vi "Test Read-Write Control.vi"(8 "error in (no error)":errorcluster) -> (0 "error out":errorcluster, 3 "Pass?":bool)   [LabVIEW 2020]
uses:
  G-Unicode/Types/UTF-8 String/UTF-8 String.lvclass/UTF-8 String.ctl
  d7f44957-dd1e-4aab-aae7-486b9bf0438c.vi
  1da8a88b-ae4e-476f-a58c-12139bd44ca5.vi
  11ce0e2c-e1a8-46a3-af78-7df26efc8245.vi
  3b8e0032-af78-4c0b-9bbb-79828ff8a6dd.vi
  70f15325-3570-4740-90b7-b159886a8434.vi
  c5b5f753-7993-4590-ab7a-38cd070e680f.vi
  1ceb00d4-36f5-49cb-928e-534e3e1f0591.vi
  1e068905-1677-418d-bf6d-609c6dcf122f.vi
  d87d6912-68ee-4c4f-8e1f-9eaf2c3e8737.vi
  8bfd12a5-a12f-46b2-9c2c-ba6b48562335.vi
  faa5ed0a-1e2a-49a9-b47c-7d87d0d78869.vi
  b51df372-b908-46a9-9cd9-1bce9bcba761.vi
  c50d1312-50c6-48d3-b875-d8e2e1e6006d.vi
  0f0a57d2-251a-4010-ac87-403ca3d19de3.vi
  3f50c59c-438d-4159-8265-e7e5e4819d1d.vi
  63b695b2-ee1d-4cc0-8b09-8d83892ddc19.vi
  a0d048c9-5e62-40e8-86eb-582b39f8129a.vi
  f481c7ac-37a4-4879-9d59-93dd94c77838.vi
  a84f4c8b-19ca-4313-b3c0-0071757116b8.vi
  daac9e31-94d2-45d0-adb4-e535b058ebe1.vi
  2abff34c-ba54-40bb-bfb0-e7a9eb1a66c8.vi
  258a67cf-78bc-49d9-a232-fa9eda3d4c17.vi
  843d702d-5434-496e-8b84-06685370aefe.vi
  b9bba32d-5ca2-4258-b841-0da24b58b874.vi
  aa946967-5c50-4c02-a82c-9d1d96941c38.vi
  74cd828c-e59a-47d5-9363-431a13b30ca9.vi
  4c20338b-6e60-4a75-91ad-9e96f58f92b0.vi
  d7f44957-dd1e-4aab-aae7-486b9bf0438c.vi/5206cb6b-04fb-41f5-a37e-29c14f142303.vi
  1da8a88b-ae4e-476f-a58c-12139bd44ca5.vi/394fe735-5a0a-4c6e-b10c-ef5f4bad8cdd.vi
  1da8a88b-ae4e-476f-a58c-12139bd44ca5.vi/c6ff4536-5c5f-4898-b0f4-ba79e0235d06.vi
  11ce0e2c-e1a8-46a3-af78-7df26efc8245.vi/3a31b270-3bb6-4c58-a256-c5fcc2c98f09.vi
  11ce0e2c-e1a8-46a3-af78-7df26efc8245.vi/0ec5df2d-ef9b-4f84-a6a8-ffcedd45c4dc.vi
  3b8e0032-af78-4c0b-9bbb-79828ff8a6dd.vi/5206cb6b-04fb-41f5-a37e-29c14f142303.vi
  70f15325-3570-4740-90b7-b159886a8434.vi/394fe735-5a0a-4c6e-b10c-ef5f4bad8cdd.vi
  70f15325-3570-4740-90b7-b159886a8434.vi/c6ff4536-5c5f-4898-b0f4-ba79e0235d06.vi
  c5b5f753-7993-4590-ab7a-38cd070e680f.vi/3a31b270-3bb6-4c58-a256-c5fcc2c98f09.vi
  c5b5f753-7993-4590-ab7a-38cd070e680f.vi/0ec5df2d-ef9b-4f84-a6a8-ffcedd45c4dc.vi
  1ceb00d4-36f5-49cb-928e-534e3e1f0591.vi/5206cb6b-04fb-41f5-a37e-29c14f142303.vi
  1e068905-1677-418d-bf6d-609c6dcf122f.vi/394fe735-5a0a-4c6e-b10c-ef5f4bad8cdd.vi
  1e068905-1677-418d-bf6d-609c6dcf122f.vi/c6ff4536-5c5f-4898-b0f4-ba79e0235d06.vi
  d87d6912-68ee-4c4f-8e1f-9eaf2c3e8737.vi/3a31b270-3bb6-4c58-a256-c5fcc2c98f09.vi
  d87d6912-68ee-4c4f-8e1f-9eaf2c3e8737.vi/0ec5df2d-ef9b-4f84-a6a8-ffcedd45c4dc.vi
  8bfd12a5-a12f-46b2-9c2c-ba6b48562335.vi/5206cb6b-04fb-41f5-a37e-29c14f142303.vi
  faa5ed0a-1e2a-49a9-b47c-7d87d0d78869.vi/394fe735-5a0a-4c6e-b10c-ef5f4bad8cdd.vi
  faa5ed0a-1e2a-49a9-b47c-7d87d0d78869.vi/c6ff4536-5c5f-4898-b0f4-ba79e0235d06.vi
  b51df372-b908-46a9-9cd9-1bce9bcba761.vi/3a31b270-3bb6-4c58-a256-c5fcc2c98f09.vi
  b51df372-b908-46a9-9cd9-1bce9bcba761.vi/0ec5df2d-ef9b-4f84-a6a8-ffcedd45c4dc.vi
  c50d1312-50c6-48d3-b875-d8e2e1e6006d.vi/5206cb6b-04fb-41f5-a37e-29c14f142303.vi
  0f0a57d2-251a-4010-ac87-403ca3d19de3.vi/394fe735-5a0a-4c6e-b10c-ef5f4bad8cdd.vi
  0f0a57d2-251a-4010-ac87-403ca3d19de3.vi/c6ff4536-5c5f-4898-b0f4-ba79e0235d06.vi
  3f50c59c-438d-4159-8265-e7e5e4819d1d.vi/3a31b270-3bb6-4c58-a256-c5fcc2c98f09.vi
  3f50c59c-438d-4159-8265-e7e5e4819d1d.vi/0ec5df2d-ef9b-4f84-a6a8-ffcedd45c4dc.vi
  63b695b2-ee1d-4cc0-8b09-8d83892ddc19.vi/5206cb6b-04fb-41f5-a37e-29c14f142303.vi
  a0d048c9-5e62-40e8-86eb-582b39f8129a.vi/394fe735-5a0a-4c6e-b10c-ef5f4bad8cdd.vi
  a0d048c9-5e62-40e8-86eb-582b39f8129a.vi/c6ff4536-5c5f-4898-b0f4-ba79e0235d06.vi
  f481c7ac-37a4-4879-9d59-93dd94c77838.vi/3a31b270-3bb6-4c58-a256-c5fcc2c98f09.vi
  f481c7ac-37a4-4879-9d59-93dd94c77838.vi/0ec5df2d-ef9b-4f84-a6a8-ffcedd45c4dc.vi
  a84f4c8b-19ca-4313-b3c0-0071757116b8.vi/5206cb6b-04fb-41f5-a37e-29c14f142303.vi
  daac9e31-94d2-45d0-adb4-e535b058ebe1.vi/394fe735-5a0a-4c6e-b10c-ef5f4bad8cdd.vi
  daac9e31-94d2-45d0-adb4-e535b058ebe1.vi/c6ff4536-5c5f-4898-b0f4-ba79e0235d06.vi
  2abff34c-ba54-40bb-bfb0-e7a9eb1a66c8.vi/3a31b270-3bb6-4c58-a256-c5fcc2c98f09.vi
  2abff34c-ba54-40bb-bfb0-e7a9eb1a66c8.vi/0ec5df2d-ef9b-4f84-a6a8-ffcedd45c4dc.vi
  258a67cf-78bc-49d9-a232-fa9eda3d4c17.vi/5206cb6b-04fb-41f5-a37e-29c14f142303.vi
  843d702d-5434-496e-8b84-06685370aefe.vi/394fe735-5a0a-4c6e-b10c-ef5f4bad8cdd.vi
  843d702d-5434-496e-8b84-06685370aefe.vi/c6ff4536-5c5f-4898-b0f4-ba79e0235d06.vi
  b9bba32d-5ca2-4258-b841-0da24b58b874.vi/3a31b270-3bb6-4c58-a256-c5fcc2c98f09.vi
  b9bba32d-5ca2-4258-b841-0da24b58b874.vi/0ec5df2d-ef9b-4f84-a6a8-ffcedd45c4dc.vi
  aa946967-5c50-4c02-a82c-9d1d96941c38.vi/5206cb6b-04fb-41f5-a37e-29c14f142303.vi
  74cd828c-e59a-47d5-9363-431a13b30ca9.vi/394fe735-5a0a-4c6e-b10c-ef5f4bad8cdd.vi
  74cd828c-e59a-47d5-9363-431a13b30ca9.vi/c6ff4536-5c5f-4898-b0f4-ba79e0235d06.vi
  4c20338b-6e60-4a75-91ad-9e96f58f92b0.vi/3a31b270-3bb6-4c58-a256-c5fcc2c98f09.vi
  4c20338b-6e60-4a75-91ad-9e96f58f92b0.vi/0ec5df2d-ef9b-4f84-a6a8-ffcedd45c4dc.vi
  G-Unicode/Private/Conversion/Text as Encoded String.vi
  G-Unicode/Private/Conversion/Polymorphic VIs/Text as Encoded String (UTF-8 String).vi
  G-Unicode/Private/Conversion/String as UTF-8 String.vi
  G-Unicode/Private/Conversion/Polymorphic VIs/String as UTF-8 String (LabVIEW String).vi
  G-Unicode/Types/UTF-8 String/Read Encoded UTF-8 String.vi
  G-Unicode/Types/UTF-8 String/New UTF-8 String.vi
  G-Unicode/Private/Conversion/Text to UTF-8.vi
  G-Unicode/Private/Conversion/Polymorphic VIs/Text to UTF-8 (LabVIEW String).vi
  G-Unicode/Private/Conversion/Encoded UTF-8 String to Encoded UTF-16LE String.vi
  G-Unicode/Private/User Interface/Write String.vi
  G-Unicode/Private/User Interface/Read String.vi
  G-Unicode/Unicode/Detect String Encoding.vi
  G-Unicode/Private/Conversion/Encoded UTF-16LE String to Encoded UTF-8 String.vi
  G-Unicode/Private/User Interface/Write String Array (1D).vi
  G-Unicode/Private/User Interface/Read String Array (1D).vi
  G-Unicode/Private/User Interface/Write String Array (2D).vi
  G-Unicode/Private/User Interface/Read String Array (2D).vi
  G-Unicode/Private/User Interface/Write Ring Control.vi
  G-Unicode/Private/User Interface/Read Ring Control.vi
  G-Unicode/Private/User Interface/Write MultCol Listbox Data.vi
  G-Unicode/Private/User Interface/Read MultCol Listbox Data.vi
  G-Unicode/Private/User Interface/Write Listbox Data.vi
  G-Unicode/Private/User Interface/Read Listbox Data.vi
  G-Unicode/Private/User Interface/Write Table Data.vi
  G-Unicode/Private/User Interface/Read Table Data.vi
  G-Unicode/Private/User Interface/Write Tab Control.vi
  G-Unicode/Private/User Interface/Read Tab Control.vi
  G-Unicode/Types/UTF-8 String/UTF-8 String.lvclass
panel:
  in  "Tab Control":enum32{"Page 1", "Page 2", "Page 3", "Page 4"}(tab)
  in  "Multicolumn Listbox":i32(listbox)
  in  "Listbox":i32(listbox)
  in  "Table Control":string[][](table)
  in  "Menu Ring":u16(ring)
  in  "Text Ring":u16(ring)
  in  "String Array (2D)":string[][](array[string])
  in  "String Array (1D)":string[](array[string])
  in  "String":string
  # "Note the dropdowns for the ring controls aren't rendered correctly, but when selected it looks OK."
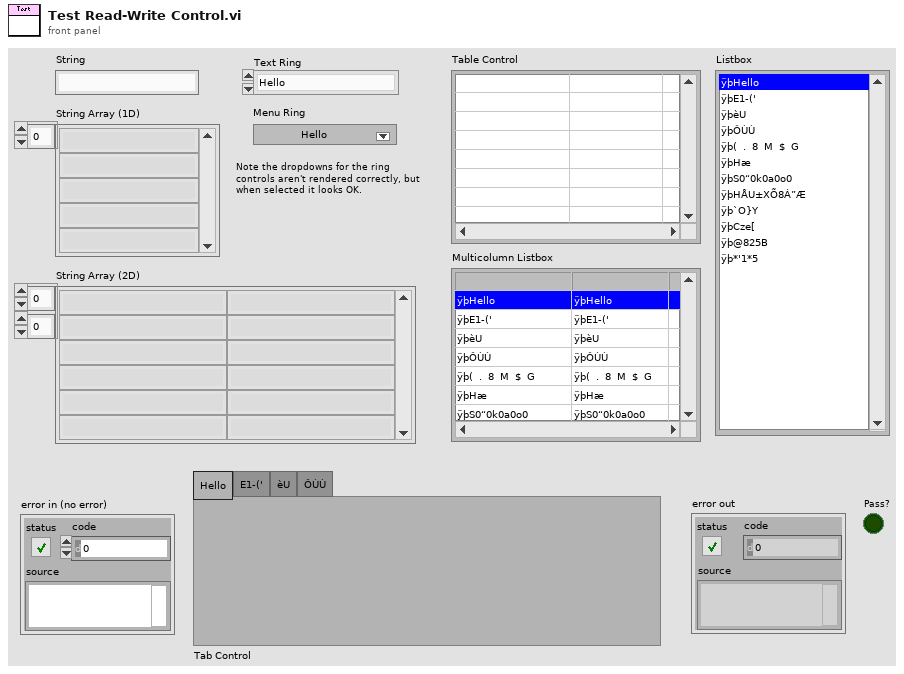
[diagram p1: front panel]
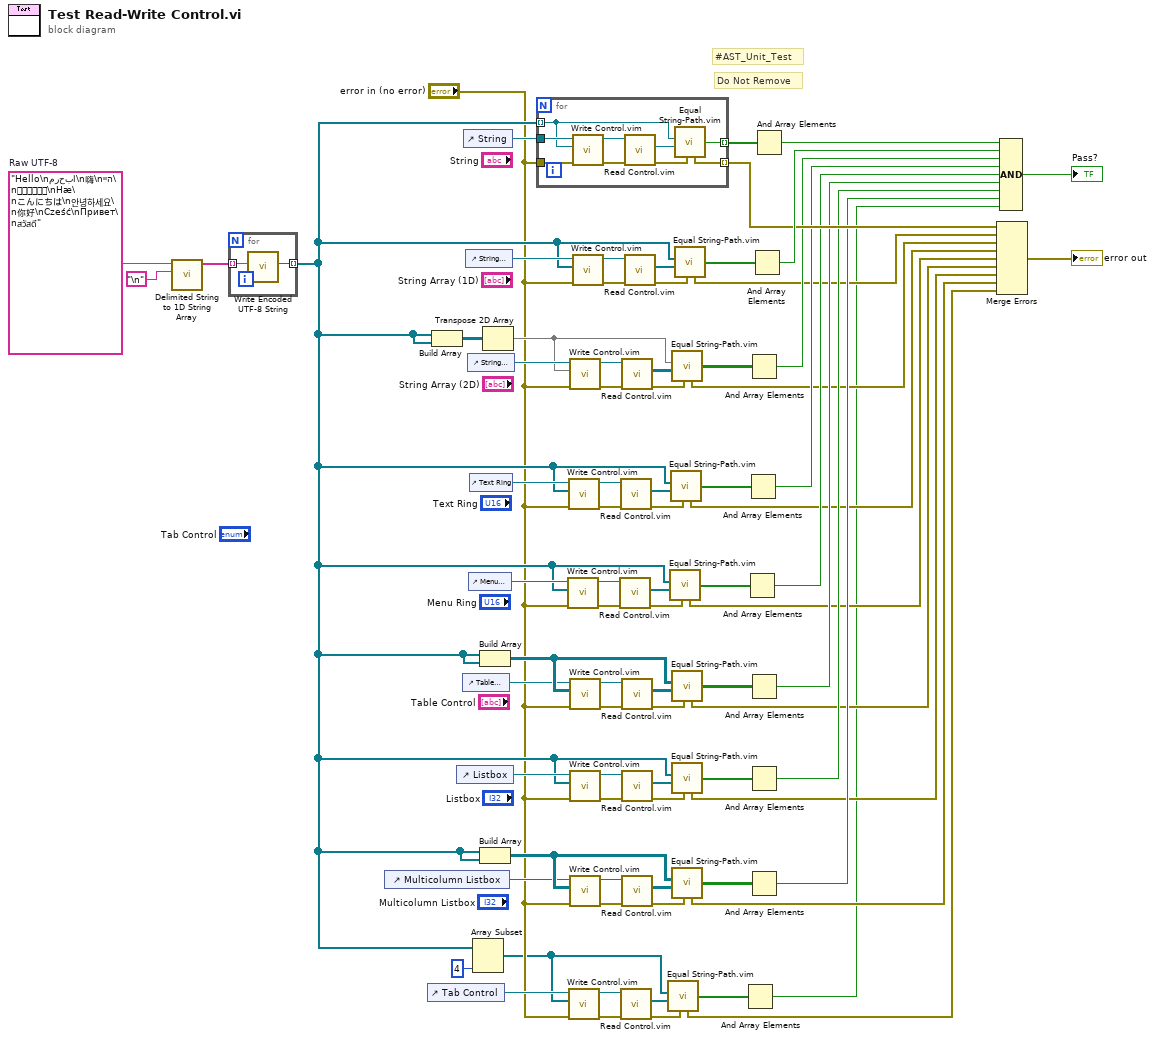
[diagram p0: block diagram]
diagram:
  w80 = "Hello\nمرحبا\n嗨\nהיי\nनमस्ते\nHæ\nこんにちは\n안녕하세요\n你好\nCześć\nПривет\nสวัสดี"  # Raw UTF-8
  # "Do Not Remove"
  # "#AST_Unit_Test"
  n1 = call <vilib>:"Delimited String to 1D String Array.vi"("delimiter"="\n", "delimited string"=w80) -> ("string array"=w79:string[])  [unwired: 9 in]
  n2 = for {
    tunnel: w79 -> [w83] mode=indexing
    tunnel: [w82] -> w12 mode=indexing
    n3 = call "Write Encoded UTF-8 String.vi"("Encoded UTF-8 String"=w83) -> ("UTF-8 String"=w82:refnum<class "UTF-8 String.lvclass">)  [unwired: 10 in]
  }
  n4 = control-ref of="Multicolumn Listbox"() -> (w29:refnum<vi>)
  n5 = control-ref of="Tab Control"() -> (w10:refnum<vi>)
  n6 = Build Array(w12, w12) -> (w62:refnum<class "UTF-8 String.lvclass">[][])
  n7 = control-ref of="Listbox"() -> (w36:refnum<vi>)
  n8 = control-ref of="Table Control"() -> (w42:refnum<vi>)
  n9 = control-ref of="String"() -> (w78:refnum<vi>)
  n10 = control-ref of="String Array (1D)"() -> (w13:refnum<vi>)
  n11 = control-ref of="String Array (2D)"() -> (w63:refnum<vi>)
  n12 = control-ref of="Menu Ring"() -> (w50:refnum<vi>)
  n13 = control-ref of="Text Ring"() -> (w55:refnum<vi>)
  n14 = Array Subset(array=w12, length=4) -> (w6:refnum<class "UTF-8 String.lvclass">[])  [unwired: 1 in]
  n15 = Build Array(w12, w12) -> (w43:refnum<class "UTF-8 String.lvclass">[][])
  n16 = Build Array(w12, w12) -> (w34:refnum<class "UTF-8 String.lvclass">[][])
  n17 = Transpose 2D Array(2D array=w62) -> (transposed array=w60:refnum<class "UTF-8 String.lvclass">[][])
  n18 = for {
    tunnel: w78 -> [w91]
    tunnel: w12 -> [w84] mode=indexing
    tunnel: "error in (no error)" -> [w90]
    tunnel: [w85] -> w68 mode=indexing
    tunnel: [w89] -> w77 mode=indexing
    n19 = call "Write Control.vim"("error in"=w90, "Text"=w84, "Control Ref"=w91) -> ("error out"=w87:errorcluster, "Control Ref dup"=w88:refnum<vi>)  [unwired: 7 in]
    n20 = call "Read Control.vim"("error in"=w87, "Control Ref"=w88) -> ("error out"=w86:errorcluster, "UTF-8 String"=w92:refnum<class "UTF-8 String.lvclass">)  [unwired: 7 in, 1 out]
    n21 = call "Equal String-Path.vim"("error in"=w86, "y"=w92, "x"=w84) -> ("error out"=w85:errorcluster, "Equal?"=w89:bool)  [unwired: 6 in]
  }
  n22 = call "Write Control.vim"("error in"="error in (no error)", "Text"=w12, "Control Ref"=w50) -> ("error out"=w53:errorcluster, "Control Ref dup"=w54:refnum<vi>)  [unwired: 7 in]
  n23 = call "Write Control.vim"("error in"="error in (no error)", "Text"=w12, "Control Ref"=w55) -> ("error out"=w57:errorcluster, "Control Ref dup"=w56:refnum<vi>)  [unwired: 7 in]
  n24 = call "Write Control.vim"("error in"="error in (no error)", "Text"=w6, "Control Ref"=w10) -> ("error out"=w8:errorcluster, "Control Ref dup"=w1:refnum<vi>)  [unwired: 7 in]
  n25 = call "Write Control.vim"("error in"="error in (no error)", "Text"=w60, "Control Ref"=w63) -> ("error out"=w66:errorcluster, "Control Ref dup"=w64:refnum<vi>)  [unwired: 7 in]
  n26 = call "Write Control.vim"("error in"="error in (no error)", "Text"=w43, "Control Ref"=w42) -> ("error out"=w45:errorcluster, "Control Ref dup"=w47:refnum<vi>)  [unwired: 7 in]
  n27 = call "Write Control.vim"("error in"="error in (no error)", "Text"=w12, "Control Ref"=w36) -> ("error out"=w38:errorcluster, "Control Ref dup"=w37:refnum<vi>)  [unwired: 7 in]
  n28 = call "Write Control.vim"("error in"="error in (no error)", "Text"=w34, "Control Ref"=w29) -> ("error out"=w32:errorcluster, "Control Ref dup"=w30:refnum<vi>)  [unwired: 7 in]
  n29 = call "Write Control.vim"("error in"="error in (no error)", "Text"=w12, "Control Ref"=w13) -> ("error out"=w71:errorcluster, "Control Ref dup"=w73:refnum<vi>)  [unwired: 7 in]
  n30 = call "Read Control.vim"("error in"=w53, "Control Ref"=w54) -> ("error out"=w19:errorcluster, "UTF-8 String"=w52:refnum<class "UTF-8 String.lvclass">[])  [unwired: 7 in, 1 out]
  n31 = call "Read Control.vim"("error in"=w57, "Control Ref"=w56) -> ("error out"=w21:errorcluster, "UTF-8 String"=w58:refnum<class "UTF-8 String.lvclass">[])  [unwired: 7 in, 1 out]
  n32 = call "Read Control.vim"("error in"=w8, "Control Ref"=w1) -> ("error out"=w5:errorcluster, "UTF-8 String"=w7:refnum<class "UTF-8 String.lvclass">[])  [unwired: 7 in, 1 out]
  n33 = call "Read Control.vim"("error in"=w66, "Control Ref"=w64) -> ("error out"=w23:errorcluster, "UTF-8 String"=w65:refnum<class "UTF-8 String.lvclass">[][])  [unwired: 7 in, 1 out]
  n34 = call "Read Control.vim"("error in"=w45, "Control Ref"=w47) -> ("error out"=w17:errorcluster, "UTF-8 String"=w46:refnum<class "UTF-8 String.lvclass">[][])  [unwired: 7 in, 1 out]
  n35 = call "Read Control.vim"("error in"=w38, "Control Ref"=w37) -> ("error out"=w15:errorcluster, "UTF-8 String"=w39:refnum<class "UTF-8 String.lvclass">[])  [unwired: 7 in, 1 out]
  n36 = call "Read Control.vim"("error in"=w32, "Control Ref"=w30) -> ("error out"=w27:errorcluster, "UTF-8 String"=w31:refnum<class "UTF-8 String.lvclass">[][])  [unwired: 7 in, 1 out]
  n37 = call "Read Control.vim"("error in"=w71, "Control Ref"=w73) -> ("error out"=w25:errorcluster, "UTF-8 String"=w72:refnum<class "UTF-8 String.lvclass">[])  [unwired: 7 in, 1 out]
  n38 = call "Equal String-Path.vim"("error in"=w5, "y"=w7, "x"=w6) -> ("error out"=w2:errorcluster, "Equal?"=w4:bool[])  [unwired: 6 in]
  n39 = call "Equal String-Path.vim"("error in"=w19, "y"=w52, "x"=w12) -> ("error out"=w18:errorcluster, "Equal?"=w51:bool[])  [unwired: 6 in]
  n40 = call "Equal String-Path.vim"("error in"=w21, "y"=w58, "x"=w12) -> ("error out"=w20:errorcluster, "Equal?"=w59:bool[])  [unwired: 6 in]
  n41 = call "Equal String-Path.vim"("error in"=w23, "y"=w65, "x"=w60) -> ("error out"=w22:errorcluster, "Equal?"=w67:bool[][])  [unwired: 6 in]
  n42 = call "Equal String-Path.vim"("error in"=w17, "y"=w46, "x"=w43) -> ("error out"=w16:errorcluster, "Equal?"=w44:bool[][])  [unwired: 6 in]
  n43 = call "Equal String-Path.vim"("error in"=w15, "y"=w39, "x"=w12) -> ("error out"=w14:errorcluster, "Equal?"=w40:bool[])  [unwired: 6 in]
  n44 = call "Equal String-Path.vim"("error in"=w27, "y"=w31, "x"=w34) -> ("error out"=w26:errorcluster, "Equal?"=w33:bool[][])  [unwired: 6 in]
  n45 = call "Equal String-Path.vim"("error in"=w25, "y"=w72, "x"=w12) -> ("error out"=w24:errorcluster, "Equal?"=w70:bool[])  [unwired: 6 in]
  n46 = And Array Elements(Boolean array=w4) -> (logical AND=w3:bool)
  n47 = And Array Elements(Boolean array=w51) -> (logical AND=w48:bool)
  n48 = And Array Elements(Boolean array=w59) -> (logical AND=w49:bool)
  n49 = And Array Elements(Boolean array=w67) -> (logical AND=w61:bool)
  n50 = And Array Elements(Boolean array=w44) -> (logical AND=w41:bool)
  n51 = And Array Elements(Boolean array=w40) -> (logical AND=w35:bool)
  n52 = And Array Elements(Boolean array=w33) -> (logical AND=w28:bool)
  n53 = And Array Elements(Boolean array=w70) -> (logical AND=w69:bool)
  n54 = And Array Elements(Boolean array=w77) -> (logical AND=w76:bool)
  n55 = Merge Errors(w68, w24, w22, w20, w18, w16, w14, w26, w2) -> (→"error out":errorcluster)
  n56 = Compound Arithmetic op=AND(w76, w69, w61, w49, w48, w41, w35, w28, w3) -> (→"Pass?":bool)
